vi "Insert table - 1.vi"() -> ()   [LabVIEW 2015]
uses:
  <vilib>/Platform/TimedLoop/XDataNode/timing_clust.ctl
  <vilib>/Platform/TimedLoop/XDataNode/nitl_modes.ctl
  <vilib>/Platform/TimedLoop/XDataNode/wakeup.ctl
  <vilib>/addons/database/Connection.llb/DB Tools Open Connec (Path).vi
  <vilib>/platform/TimedLoop/XDataNode/XDataNode.xnode
  <vilib>/addons/database/NI_Database_API.lvlib
  <vilib>/Platform/TimedLoop/XDataNode/XDNodeRunTimeDep.lvlib
panel:
  out "Time":u32
  out "Counter":i32
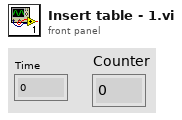
[diagram p1: front panel]
types:
  T1 = typedef "NI_Database_API.lvlib/Conn ObjectReference.ctl" = refnum<k1>
  T2 = typedef "XDNodeRunTimeDep.lvlib/timing_clust.ctl" = cluster{"Expected End [f-1]":u64, "Actual End [f-1]":u64, "Finished Late? [f-1]":bool, "Expected End [i-1]":u64, "Actual End [i-1]":u64, "Finished Late? [i-1]":bool, "Expected Start [i]":u64, "Actual Start [i]":u64, "Expected Start [f]":u64, "Actual Start [f]":u64, "Source Name":string, "Structure Name":string, "Period":i64, "Deadline":i64, "Offset":i64, "Start":i64, "Priority":i32, "Timeout":i32, "Mode":T3, "Wakeup Reason":T4, "Error":errorcluster, "Source Type":string, "Secondary Source Type":string, "Global End Time":u64, "Global Start Time":u64, "Frame Duration":u64, "Iteration Duration":u64, "Assigned CPU":i32, "I/O Scan Engine Mode":u32}
  T3 = typedef "XDNodeRunTimeDep.lvlib/nitl_modes.ctl" = enum32{"No Change", "Process missed periods, maintain original phase", "Discard missed periods, maintain original phase", "Process missed periods, ignore original phase", "Discard missed periods, ignore original phase"}
  T4 = typedef "XDNodeRunTimeDep.lvlib/wakeup.ctl" = enum32{"Normal", "Aborted", "Asynchronous wakeup", "Timing source error", "Timed loop error", "Timeout"}
  T5 = cluster{"Numeric":i32, "Numeric":i32, "Numeric":i32, "Numeric":i32, "Numeric":i32, "Numeric":i32, "Numeric":i32, "Numeric":i32, "Numeric":i32, "Numeric":i32, "Numeric":i32, "Numeric":i32, "Numeric":i32, "Numeric":i32, "Numeric":i32, "Numeric":i32, "Numeric":i32, "Numeric":i32, "Numeric":i32, "Numeric":i32, "Numeric":i32, "Numeric":i32, "Numeric":i32, "Numeric":i32, "Numeric":i32, "Numeric":i32, "Numeric":i32, "Numeric":i32, "Numeric":i32, "Numeric":i32, "Numeric":i32, "Numeric":i32, "Numeric":i32, "Numeric":i32, "Numeric":i32, "Numeric":i32, "Numeric":i32, "Numeric":i32, "Numeric":i32, "Numeric":i32, "Numeric":i32, "Numeric":i32, "Numeric":i32, "Numeric":i32, "Numeric":i32, "Numeric":i32, "Numeric":i32, "Numeric":i32, "Numeric":i32, "Numeric":i32, "Numeric":i32, "Numeric":i32, "Numeric":i32, "Numeric":i32, "Numeric":i32, "Numeric":i32, "Numeric":i32, "Numeric":i32, "Numeric":i32, "Numeric":i32, "Numeric":i32, "Numeric":i32, "Numeric":i32, "Numeric":i32, "Numeric":i32, "Numeric":i32, "Numeric":i32, "Numeric":i32, "Numeric":i32, "Numeric":i32, "Numeric":i32, "Numeric":i32, "Numeric":i32, "Numeric":i32, "Numeric":i32, "Numeric":i32, "Numeric":i32, "Numeric":i32, "Numeric":i32, "Numeric":i32, "Numeric":i32, "Numeric":i32, "Numeric":i32, "Numeric":i32, "Numeric":i32, "Numeric":i32, "Numeric":i32, "Numeric":i32, "Numeric":i32, "Numeric":i32, "Numeric":i32, "Numeric":i32, "Numeric":i32, "Numeric":i32, "Numeric":i32, "Numeric":i32, "Numeric":i32, "Numeric":i32, "Numeric":i32, "Numeric":i32}
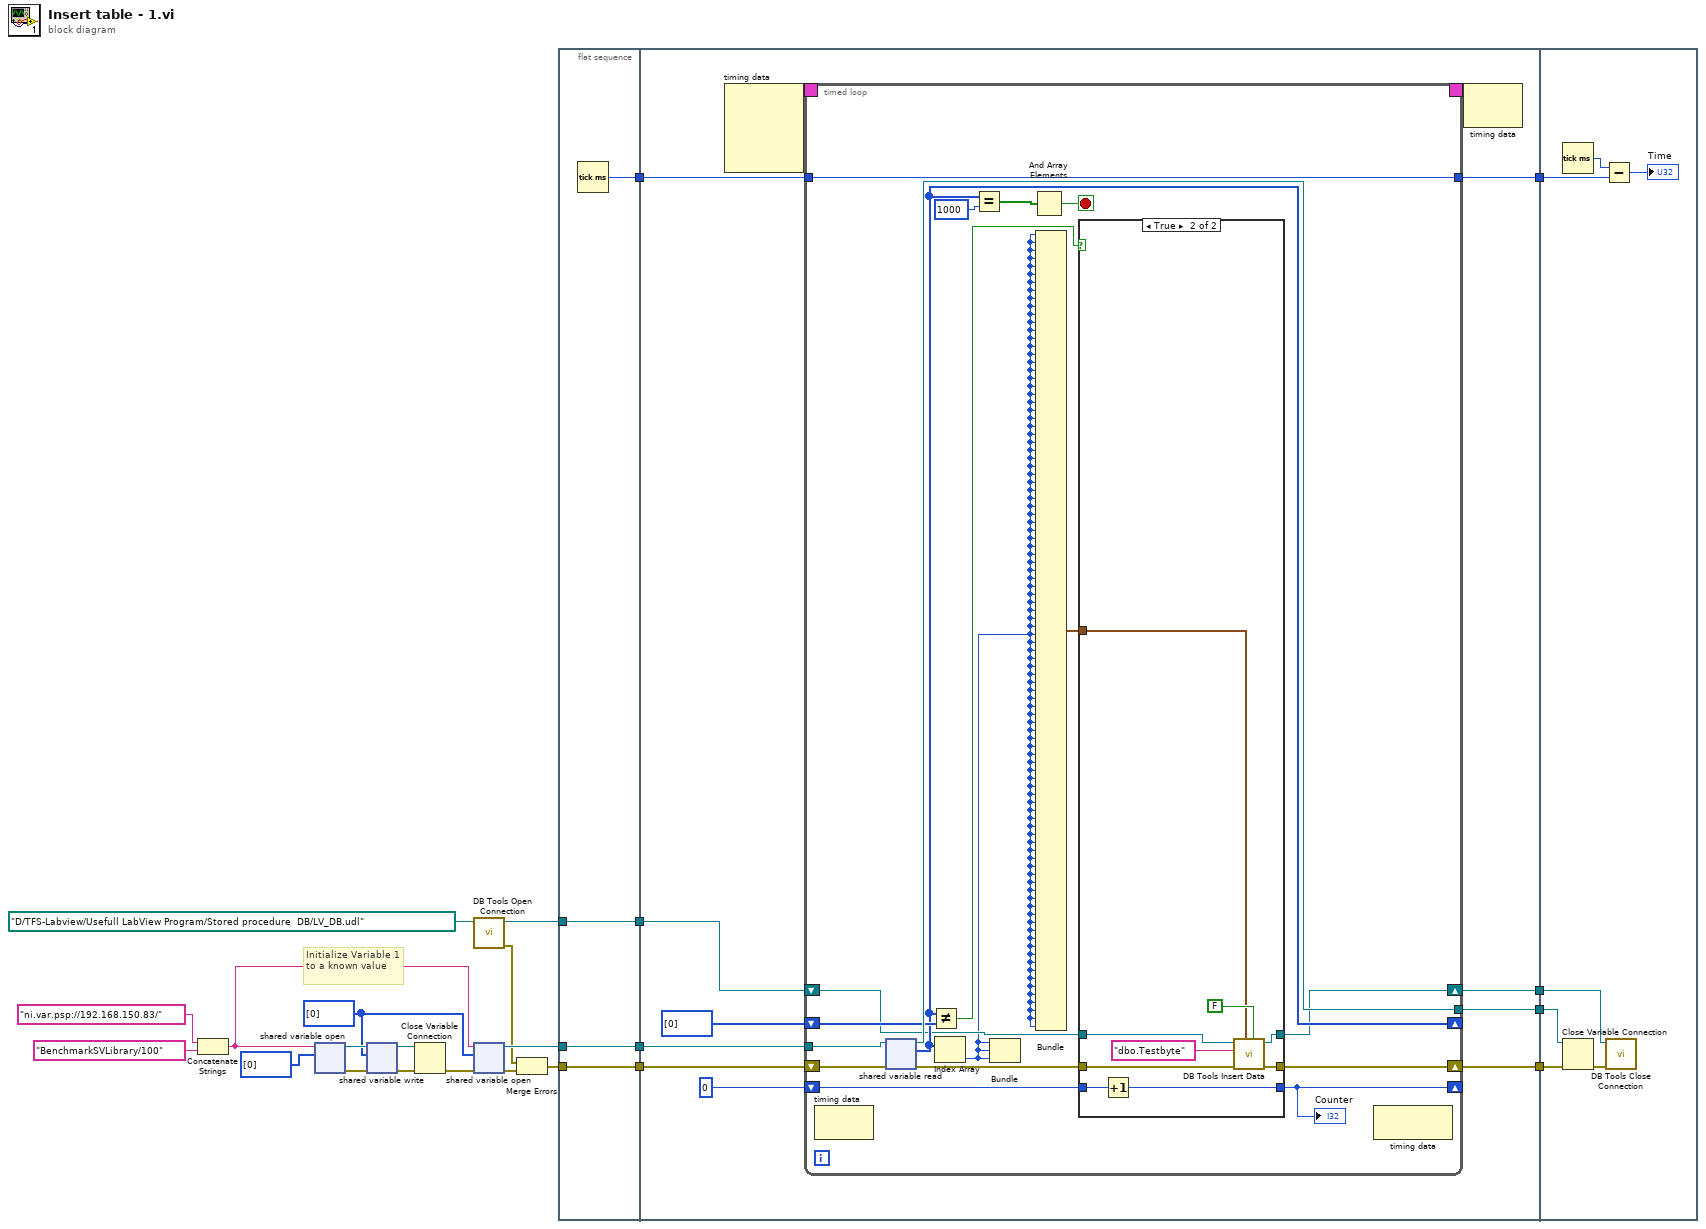
[diagram p0: block diagram]
diagram:
  w8 = i32[] [0] ("1000 Byte 3")
  # "Initialize Variable 1 to a known value"
  n1 = Concatenate Strings("ni.var.psp://192.168.150.83/" ("string"), "BenchmarkSVLibrary/100") -> (w7:string)
  n2 = shared-variable-open(w7, i32[] [0] ("appended array")) -> (w15:refnum<k21>, w13:errorcluster)  [unwired: 2 in]
  n3 = shared-variable-write(w15, w13, w8) -> (w14:refnum<k21>, w12:errorcluster)
  n4 = Close Variable Connection(8:w12, 11:w14) -> (0:w9:errorcluster)
  n5 = call-poly <vilib>:"DB Tools Open Connection.vi"("connection information"=path "D:/TFS-Labview/Usefull LabView Program/Stored procedure  DB/LV_DB.udl") -> ("error out"=w3:errorcluster, "connection reference"=w5:T1)  [unwired: 7 in]
  n6 = shared-variable-open(w7, w9, w8) -> (w17:refnum<k21>, w2:errorcluster)  [unwired: 1 in]
  n7 = Merge Errors(w3, w2) -> (w1:errorcluster)
  n8 = flat-sequence {
    tunnel: w17 -> [w27]
    tunnel: w1 -> [w28]
    tunnel: [w28] -> w23
    tunnel: [w27] -> w22
    tunnel: [w26] -> w21
    tunnel: [w25] -> w6
    tunnel: w5 -> [w25]
    tunnel: [w37] -> w20
    tunnel: [w36] -> w19
    tunnel: [w34] -> w18
    tunnel: w23 -> [w40]
    tunnel: w22 -> [w39]
    tunnel: w21 -> [w35]
    tunnel: w6 -> [w30]
    tunnel: [w29] -> w4
    tunnel: w20 -> [w78]
    tunnel: w19 -> [w77]
    tunnel: w18 -> [w79]
    tunnel: w4 -> [w76]
    frame #0 {
      n9 = Tick Count (ms)() -> (millisecond timer value=w26:u32)
    }
    frame #1 {
      n10 = node-c288() -> (w32:T2)  [unwired: 4 in]
      n11 = timed-loop {
        shift-right: [w47] -> _
        shift-left: i32[] [0] ("1000 Byte 3") -> [w51]
        shift-right: [w45] -> w37
        shift-left: w40 -> [w56]
        shift-right: [w52] -> _
        shift-left: 0 -> [w58]
        tunnel: w39 -> [w57]
        tunnel: [w55] -> w36
        tunnel: [w53] -> w34
        tunnel: w35 -> [w53]
        timing: w32 -> [_]
        timing-out: [_] -> w31
        shift-right: [w43] -> w29
        shift-left: w30 -> [w44]
        stop <- w49 stop-if-true
        n12 = node-c288() -> ()  [unwired: 1 in, 1 out]
        n13 = shared-variable-read(w57, w56) -> (w55:refnum<k21>, w46:errorcluster, w47:i32[])  [unwired: 1 out]
        n14 = Not Equal?(x=w47, y=w51) -> (x != y?=w54:bool)
        n15 = Index Array(array=w47) -> (element=w41:i32)  [unwired: 1 in]
        n16 = Equal?(x=w47, y=1000 ("Numeric")) -> (x = y?=w48:bool[])
        n17 = Bundle("Numeric"=w41, "Numeric"=w41, "Numeric"=w41) -> ()  [unwired: 1 in, 1 out]
        n18 = And Array Elements(Boolean array=w48) -> (logical AND=w49:bool)
        n19 = Bundle("Numeric"=w41, "Numeric"=w41, "Numeric"=w41, "Numeric"=w41, "Numeric"=w41, "Numeric"=w41, "Numeric"=w41, "Numeric"=w41, "Numeric"=w41, "Numeric"=w41, "Numeric"=w41, "Numeric"=w41, "Numeric"=w41, "Numeric"=w41, "Numeric"=w41, "Numeric"=w41, "Numeric"=w41, "Numeric"=w41, "Numeric"=w41, "Numeric"=w41, "Numeric"=w41, "Numeric"=w41, "Numeric"=w41, "Numeric"=w41, "Numeric"=w41, "Numeric"=w41, "Numeric"=w41, "Numeric"=w41, "Numeric"=w41, "Numeric"=w41, "Numeric"=w41, "Numeric"=w41, "Numeric"=w41, "Numeric"=w41, "Numeric"=w41, "Numeric"=w41, "Numeric"=w41, "Numeric"=w41, "Numeric"=w41, "Numeric"=w41, "Numeric"=w41, "Numeric"=w41, "Numeric"=w41, "Numeric"=w41, "Numeric"=w41, "Numeric"=w41, "Numeric"=w41, "Numeric"=w41, "Numeric"=w41, "Numeric"=w41, "Numeric"=w41, "Numeric"=w41, "Numeric"=w41, "Numeric"=w41, "Numeric"=w41, "Numeric"=w41, "Numeric"=w41, "Numeric"=w41, "Numeric"=w41, "Numeric"=w41, "Numeric"=w41, "Numeric"=w41, "Numeric"=w41, "Numeric"=w41, "Numeric"=w41, "Numeric"=w41, "Numeric"=w41, "Numeric"=w41, "Numeric"=w41, "Numeric"=w41, "Numeric"=w41, "Numeric"=w41, "Numeric"=w41, "Numeric"=w41, "Numeric"=w41, "Numeric"=w41, "Numeric"=w41, "Numeric"=w41, "Numeric"=w41, "Numeric"=w41, "Numeric"=w41, "Numeric"=w41, "Numeric"=w41, "Numeric"=w41, "Numeric"=w41, "Numeric"=w41, "Numeric"=w41, "Numeric"=w41, "Numeric"=w41, "Numeric"=w41, "Numeric"=w41, "Numeric"=w41, "Numeric"=w41, "Numeric"=w41, "Numeric"=w41, "Numeric"=w41, "Numeric"=w41, "Numeric"=w41, "Numeric"=w41, "Numeric"=w41) -> (w42:T5)  [unwired: 1 in]
        n20 = case shown="True" w54 {
          tunnel: w58 -> [w63 w72]
          tunnel: [w63 w71] -> w52
          tunnel: w46 -> [w62 w68]
          tunnel: [w62 w67] -> w45
          tunnel: w44 -> [w61 w66]
          tunnel: [w61 w65] -> w43
          tunnel: w42 -> [_ w64]
          frame False {
          }
          frame True {
            n21 = Increment(x=w72) -> (x+1=w71:i32)
            n22 = call <vilib>:"DB Tools Insert Data.vi"("create table? (F)"=FALSE, "data"=w64, "error in (no error)"=w68, "table"="dbo.Testbyte" ("SQL query"), "connection reference"=w66) -> ("error out"=w67:errorcluster, "connection reference out"=w65:T1)  [unwired: 5 in]
          }
        }
        "Counter" <- w52
        n23 = node-c288() -> ()  [unwired: 1 in, 1 out]
      }
      n24 = node-c288(w31) -> ()  [unwired: 1 out]
    }
    frame #2 {
      n25 = Tick Count (ms)() -> (millisecond timer value=w81:u32)
      n26 = Close Variable Connection(8:w78, 11:w77) -> (0:w75:errorcluster)
      n27 = Subtract(x=w81, y=w79) -> (x-y=→"Time":u32)
      n28 = call <vilib>:"DB Tools Close Connection.vi"("error in (no error)"=w75, "connection reference"=w76) -> ()  [unwired: 5 in, 1 out]
    }
  }
